vi "test grpc xnet.vi"() -> ()   [LabVIEW 2025]
uses:
  RPC Messages/nixnet_grpc_CreateSessionRequest.ctl
  RPC Messages/nixnet_grpc_CreateSessionRequest_mode_enum/nixnet_grpc_CreateSessionRequest_mode_enum.lvclass
  RPC Messages/nidevice_grpc_SessionInitializationBehavior.ctl
  RPC Messages/nixnet_grpc_CreateSessionMode.ctl
  RPC Messages/nixnet_grpc_CreateSessionRequest_mode_enum/nixnet_grpc_CreateSessionRequest_mode_enum.lvclass/nixnet_grpc_CreateSessionRequest_mode_enum.ctl
  RPC Messages/nixnet_grpc_ClearRequest.ctl
  RPC Messages/nidevice_grpc_Session.ctl
  RPC Messages/nixnet_grpc_SetPropertyRequest.ctl
  RPC Messages/nixnet_grpc_SetPropertyRequest_property_id_enum/nixnet_grpc_SetPropertyRequest_property_id_enum.lvclass
  RPC Messages/nixnet_grpc_SetPropertyRequest_property_value/nixnet_grpc_SetPropertyRequest_property_value.lvclass
  RPC Messages/nixnet_grpc_Property.ctl
  RPC Messages/nixnet_grpc_SetPropertyRequest_property_id_enum/nixnet_grpc_SetPropertyRequest_property_id_enum.lvclass/nixnet_grpc_SetPropertyRequest_property_id_enum.ctl
  RPC Messages/nixnet_grpc_SetPropertyRequest_property_value/nixnet_grpc_SetPropertyRequest_property_value.lvclass/nixnet_grpc_SetPropertyRequest_property_value.ctl
  RPC Messages/nixnet_grpc_ReadFrameRequest.ctl
  RPC Messages/nixnet_grpc_ReadFrameRequest_protocol_enum/nixnet_grpc_ReadFrameRequest_protocol_enum.lvclass
  RPC Messages/nixnet_grpc_ReadFrameRequest_timeout_enum/nixnet_grpc_ReadFrameRequest_timeout_enum.lvclass
  RPC Messages/nixnet_grpc_Protocol.ctl
  RPC Messages/nixnet_grpc_ReadFrameRequest_protocol_enum/nixnet_grpc_ReadFrameRequest_protocol_enum.lvclass/nixnet_grpc_ReadFrameRequest_protocol_enum.ctl
  RPC Messages/nixnet_grpc_TimeOut.ctl
  RPC Messages/nixnet_grpc_ReadFrameRequest_timeout_enum/nixnet_grpc_ReadFrameRequest_timeout_enum.lvclass/nixnet_grpc_ReadFrameRequest_timeout_enum.ctl
  RPC Messages/nixnet_grpc_FrameBufferResponse_frame/nixnet_grpc_FrameBufferResponse_frame.lvclass/nixnet_grpc_FrameBufferResponse_frame.ctl
  xnet-grpc_client.lvlib
  RPC Messages/nixnet_grpc_FrameBufferResponse_frame/nixnet_grpc_FrameBufferResponse_frame.lvclass
panel:
  out "new_session_initialized":bool
  out "create session status":i32
  out "status":i32
  out "payload":u8[](array[numeric])
  out "identifier":u32
  in  "Stop":bool
  out "error out":errorcluster
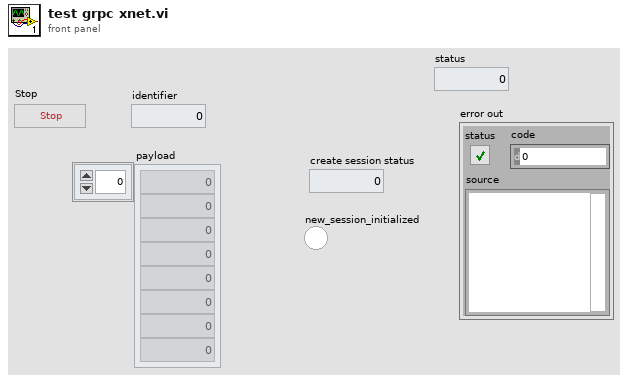
[diagram p1: front panel]
types:
  T1 = typedef "xnet-grpc_client.lvlib/nixnet_grpc_TimeOut.ctl" = enum32{"TIME_OUT_NONE", "TIME_OUT_INFINITE"}
  T2 = typedef "xnet-grpc_client.lvlib/nixnet_grpc_Protocol.ctl" = enum32{"PROTOCOL_UNSPECIFIED", "PROTOCOL_CAN", "PROTOCOL_LIN", "PROTOCOL_FLEX_RAY", "PROTOCOL_J1939", "PROTOCOL_ENET"}
  T3 = typedef "xnet-grpc_client.lvlib/nixnet_grpc_ReadFrameRequest.ctl" = cluster{"session":T4, "number_of_frames":i32, "max_payload_per_frame":u32, "nixnet_grpc_ReadFrameRequest_protocol_enum":refnum<class "nixnet_grpc_ReadFrameRequest_protocol_enum.lvclass">, "nixnet_grpc_ReadFrameRequest_timeout_enum":refnum<class "nixnet_grpc_ReadFrameRequest_timeout_enum.lvclass">}
  T4 = typedef "xnet-grpc_client.lvlib/nidevice_grpc_Session.ctl" = cluster{"name":string}
  T5 = typedef "xnet-grpc_client.lvlib/nixnet_grpc_Property.ctl" = enum32{"PROPERTY_UNSPECIFIED", "PROPERTY_SESSION_APPLICATION_PROTOCOL", "PROPERTY_SESSION_AUTO_START", "PROPERTY_SESSION_CLUSTER_NAME", "PROPERTY_SESSION_DATABASE_NAME", "PROPERTY_SESSION_ENET_FRAME_FILTER", "PROPERTY_SESSION_ENET_LOG_ERROR", "PROPERTY_SESSION_ENET_LOG_FILE", "PROPERTY_SESSION_ENET_LOG_MODE", "PROPERTY_SESSION_ENET_LOG_ENABLE_MULTIPLE_FILES", "PROPERTY_SESSION_ENET_LOG_FILE_SIZE_THRESHOLD", "PROPERTY_SESSION_ENET_LOG_OPERATION", "PROPERTY_SESSION_ENET_NUM_FRAMES_RECEIVED", "PROPERTY_SESSION_ENET_SOURCE_MAC_ADDRESS_AUTO", "PROPERTY_SESSION_INTF_BAUD_RATE_64", "PROPERTY_SESSION_INTF_ADJUST_LOCAL_TIME", "PROPERTY_SESSION_INTF_BAUD_RATE", "PROPERTY_SESSION_INTF_BUS_ERR_TO_IN_STRM", "PROPERTY_SESSION_INTF_CAN_FD_BAUD_RATE_64", "PROPERTY_SESSION_INTF_CAN_DISABLE_PROT_EXCEPTION_HANDLING", "PROPERTY_SESSION_INTF_CAN_EDGE_FILTER", "PROPERTY_SESSION_INTF_CAN_EXT_TCVR_CONFIG", "PROPERTY_SESSION_INTF_CAN_FD_BAUD_RATE", "PROPERTY_SESSION_INTF_CAN_FD_ISO_MODE", "PROPERTY_SESSION_INTF_CAN_IO_MODE", "PROPERTY_SESSION_INTF_CAN_LSTN_ONLY", "PROPERTY_SESSION_INTF_CAN_PEND_TX_ORDER", "PROPERTY_SESSION_INTF_CAN_SING_SHOT", "PROPERTY_SESSION_INTF_CAN_TERM", "PROPERTY_SESSION_INTF_CAN_TCVR_STATE", "PROPERTY_SESSION_INTF_CAN_TCVR_TYPE", "PROPERTY_SESSION_INTF_CAN_TX_IO_MODE", "PROPERTY_SESSION_INTF_CAN_TRANSMIT_PAUSE", "PROPERTY_SESSION_INTF_ECHO_TX", "PROPERTY_SESSION_INTF_ENET_EPT_RECEIVE_FILTER", "PROPERTY_SESSION_INTF_ENET_EPT_TRANSMIT_BANDWIDTH", "PROPERTY_SESSION_INTF_ENET_IPV4_ADDRESS", "PROPERTY_SESSION_INTF_ENET_JUMBO_FRAMES", "PROPERTY_SESSION_INTF_ENET_LINK_SPEED", "PROPERTY_SESSION_INTF_ENET_LINK_SPEED_CONFIGURED", "PROPERTY_SESSION_INTF_ENET_MAC_ADDRESS", "PROPERTY_SESSION_INTF_ENET_OS_NETWORK_ADAPTER_DESCRIPTION", "PROPERTY_SESSION_INTF_ENET_OS_NETWORK_ADAPTER_NAME", "PROPERTY_SESSION_INTF_ENET_OPERATIONAL_STATUS", "PROPERTY_SESSION_INTF_ENET_OUT_STRM_TIMESCALE", "PROPERTY_SESSION_INTF_ENET_PHY_POWER_MODE", "PROPERTY_SESSION_INTF_ENET_PHY_STATE", "PROPERTY_SESSION_INTF_ENET_PORT_MODE", "PROPERTY_SESSION_INTF_ENET_SIGNAL_QUALITY", "PROPERTY_SESSION_INTF_ENET_SLEEP_CAPABILITY", "PROPERTY_SESSION_INTF_ENET_STATS_COUNTER_NAMES", "PROPERTY_SESSION_INTF_ENET_STATS_COUNTER_VALUES", "PROPERTY_SESSION_INTF_ENET_STATS_RX_BAD_FRAMES", "PROPERTY_SESSION_INTF_ENET_STATS_RX_BYTES", "PROPERTY_SESSION_INTF_ENET_STATS_RX_GOOD_FRAMES", "PROPERTY_SESSION_INTF_ENET_STATS_TX_BYTES", "PROPERTY_SESSION_INTF_ENET_STATS_TX_GOOD_FRAMES", "PROPERTY_SESSION_INTF_ENET_STATS_PHY_COUNTER_NAMES", "PROPERTY_SESSION_INTF_ENET_STATS_PHY_COUNTER_VALUES", "PROPERTY_SESSION_INTF_ENET_STATS_PHY_LOW_POWER_SLEEP", "PROPERTY_SESSION_INTF_ENET_STATS_PHY_SLEEP_FAILURE", "PROPERTY_SESSION_INTF_ENET_STATS_PHY_WAKEUP_FAILURE", "PROPERTY_SESSION_INTF_ENET_STATS_PHY_WAKEUP_PULSE", "PROPERTY_SESSION_INTF_ENET_STATS_PHY_WAKEUP_REQUEST", "PROPERTY_SESSION_INTF_ENET_TIME_ADJUST_NETWORK_TIME", "PROPERTY_SESSION_INTF_ENET_TIME_BMCA_ENABLED", "PROPERTY_SESSION_INTF_ENET_TIME_CLK_ACCURACY", "PROPERTY_SESSION_INTF_ENET_TIME_CLK_CLASS", "PROPERTY_SESSION_INTF_ENET_TIME_CLK_ID", "PROPERTY_SESSION_INTF_ENET_TIME_CLK_OFFSET_VAR", "PROPERTY_SESSION_INTF_ENET_TIME_GM_CLK_ACCURACY", "PROPERTY_SESSION_INTF_ENET_TIME_GM_CLK_CLASS", "PROPERTY_SESSION_INTF_ENET_TIME_GM_CLK_ID", "PROPERTY_SESSION_INTF_ENET_TIME_GM_CLK_OFFSET_VAR", "PROPERTY_SESSION_INTF_ENET_TIME_GM_PRIORITY_1", "PROPERTY_SESSION_INTF_ENET_TIME_GM_PRIORITY_2", "PROPERTY_SESSION_INTF_ENET_TIME_OFFSET_FROM_MASTER", "PROPERTY_SESSION_INTF_ENET_TIME_PORT_AS_CAPABLE", "PROPERTY_SESSION_INTF_ENET_TIME_PORT_ANNOUNCE_RECEIPT_TIMEOUT", "PROPERTY_SESSION_INTF_ENET_TIME_PORT_ANNOUNCE_TRANSMIT_ENABLED", "PROPERTY_SESSION_INTF_ENET_TIME_PORT_LOG_ANNOUNCE_INTERVAL", "PROPERTY_SESSION_INTF_ENET_TIME_PORT_LOG_ANNOUNCE_INTERVAL_CONFIGURED", "PROPERTY_SESSION_INTF_ENET_TIME_PORT_LOG_PDELAY_INTERVAL", "PROPERTY_SESSION_INTF_ENET_TIME_PORT_LOG_PDELAY_INTERVAL_CONFIGURED", "PROPERTY_SESSION_INTF_ENET_TIME_PORT_LOG_SYNC_INTERVAL", "PROPERTY_SESSION_INTF_ENET_TIME_PORT_LOG_SYNC_INTERVAL_CONFIGURED", "PROPERTY_SESSION_INTF_ENET_TIME_PORT_PDELAY_ENABLED", "PROPERTY_SESSION_INTF_ENET_TIME_PORT_STATE", "PROPERTY_SESSION_INTF_ENET_TIME_PORT_STATE_CONFIGURED", "PROPERTY_SESSION_INTF_ENET_TIME_PORT_PROP_DELAY", "PROPERTY_SESSION_INTF_ENET_TIME_PORT_PROP_DELAY_CONFIGURED", "PROPERTY_SESSION_INTF_ENET_TIME_PORT_PROP_DELAY_THRESHOLD", "PROPERTY_SESSION_INTF_ENET_TIME_PORT_STATS_COUNTER_NAMES", "PROPERTY_SESSION_INTF_ENET_TIME_PORT_STATS_COUNTER_VALUES", "PROPERTY_SESSION_INTF_ENET_TIME_PORT_STATS_RX_ANNOUNCE", "PROPERTY_SESSION_INTF_ENET_TIME_PORT_STATS_RX_PDELAY_REQUEST", "PROPERTY_SESSION_INTF_ENET_TIME_PORT_STATS_RX_SYNC", "PROPERTY_SESSION_INTF_ENET_TIME_PORT_STATS_TX_ANNOUNCE", "PROPERTY_SESSION_INTF_ENET_TIME_PORT_STATS_TX_PDELAY_REQUEST", "PROPERTY_SESSION_INTF_ENET_TIME_PORT_STATS_TX_SYNC", "PROPERTY_SESSION_INTF_ENET_TIME_PORT_SYNC_RECEIPT_TIMEOUT", "PROPERTY_SESSION_INTF_ENET_TIME_PORT_SYNC_STATUS", "PROPERTY_SESSION_INTF_ENET_TIME_PORT_SYNCED", "PROPERTY_SESSION_INTF_ENET_TIME_PRIORITY_1", "PROPERTY_SESSION_INTF_ENET_TIME_PRIORITY_2", "PROPERTY_SESSION_INTF_ENET_TIME_PROTOCOL", "PROPERTY_SESSION_INTF_ENET_TIME_PROTOCOL_ENABLED", "PROPERTY_SESSION_INTF_ENET_TIME_STEPS_TO_GM", "PROPERTY_SESSION_INTF_ENET_TRIGGER_PPS_SYNCED", "PROPERTY_SESSION_INTF_FLEX_RAY_ACC_START_RNG", "PROPERTY_SESSION_INTF_FLEX_RAY_ALW_HLT_CLK", "PROPERTY_SESSION_INTF_FLEX_RAY_ALW_PASS_ACT", "PROPERTY_SESSION_INTF_FLEX_RAY_AUTO_ASLP_WHN_STP", "PROPERTY_SESSION_INTF_FLEX_RAY_CLST_DRIFT_DMP", "PROPERTY_SESSION_INTF_FLEX_RAY_COLDSTART", "PROPERTY_SESSION_INTF_FLEX_RAY_CONNECTED_CHS", "PROPERTY_SESSION_INTF_FLEX_RAY_DEC_CORR", "PROPERTY_SESSION_INTF_FLEX_RAY_DELAY_COMP_A", "PROPERTY_SESSION_INTF_FLEX_RAY_DELAY_COMP_B", "PROPERTY_SESSION_INTF_FLEX_RAY_KEY_SLOT_ID", "PROPERTY_SESSION_INTF_FLEX_RAY_LATEST_TX", "PROPERTY_SESSION_INTF_FLEX_RAY_LIST_TIMO", "PROPERTY_SESSION_INTF_FLEX_RAY_MAC_INIT_OFF_A", "PROPERTY_SESSION_INTF_FLEX_RAY_MAC_INIT_OFF_B", "PROPERTY_SESSION_INTF_FLEX_RAY_MAX_DRIFT", "PROPERTY_SESSION_INTF_FLEX_RAY_MIC_INIT_OFF_A", "PROPERTY_SESSION_INTF_FLEX_RAY_MIC_INIT_OFF_B", "PROPERTY_SESSION_INTF_FLEX_RAY_MICROTICK", "PROPERTY_SESSION_INTF_FLEX_RAY_NULL_TO_IN_STRM", "PROPERTY_SESSION_INTF_FLEX_RAY_OFF_CORR", "PROPERTY_SESSION_INTF_FLEX_RAY_OFF_CORR_OUT", "PROPERTY_SESSION_INTF_FLEX_RAY_RATE_CORR", "PROPERTY_SESSION_INTF_FLEX_RAY_RATE_CORR_OUT", "PROPERTY_SESSION_INTF_FLEX_RAY_SAMP_PER_MICRO", "PROPERTY_SESSION_INTF_FLEX_RAY_SING_SLOT_EN", "PROPERTY_SESSION_INTF_FLEX_RAY_SLEEP", "PROPERTY_SESSION_INTF_FLEX_RAY_STATISTICS_EN", "PROPERTY_SESSION_INTF_FLEX_RAY_SYM_TO_IN_STRM", "PROPERTY_SESSION_INTF_FLEX_RAY_SYNC_STATUS", "PROPERTY_SESSION_INTF_FLEX_RAY_SYNC_CH_A_EVEN", "PROPERTY_SESSION_INTF_FLEX_RAY_SYNC_CH_A_ODD", "PROPERTY_SESSION_INTF_FLEX_RAY_SYNC_CH_B_EVEN", "PROPERTY_SESSION_INTF_FLEX_RAY_SYNC_CH_B_ODD", "PROPERTY_SESSION_INTF_FLEX_RAY_TERM", "PROPERTY_SESSION_INTF_FLEX_RAY_WAKEUP_CH", "PROPERTY_SESSION_INTF_FLEX_RAY_WAKEUP_PTRN", "PROPERTY_SESSION_INTF_NAME", "PROPERTY_SESSION_INTF_LIN_BREAK_DELIMITER_LENGTH", "PROPERTY_SESSION_INTF_LIN_BREAK_LENGTH", "PROPERTY_SESSION_INTF_LIN_CHECKSUM_TO_IN_STRM", "PROPERTY_SESSION_INTF_LIN_DIAG_P2_MIN", "PROPERTY_SESSION_INTF_LIN_DIAG_ST_MIN", "PROPERTY_SESSION_INTF_LIN_MASTER", "PROPERTY_SESSION_INTF_LIN_NO_RESPONSE_TO_IN_STRM", "PROPERTY_SESSION_INTF_LINO_STR_SLV_RSP_LST_BY_NAD", "PROPERTY_SESSION_INTF_LIN_SCHED_NAMES", "PROPERTY_SESSION_INTF_LIN_SLEEP", "PROPERTY_SESSION_INTF_LIN_ALW_START_WO_BUS_PWR", "PROPERTY_SESSION_INTF_LIN_TERM", "PROPERTY_SESSION_INTF_OUT_STRM_LIST", "PROPERTY_SESSION_INTF_OUT_STRM_LIST_BY_ID", "PROPERTY_SESSION_INTF_OUT_STRM_TIMNG", "PROPERTY_SESSION_INTF_SRC_TERM_START_TRIGGER", "PROPERTY_SESSION_INTF_START_TRIG_TO_IN_STRM", "PROPERTY_SESSION_LIST", "PROPERTY_SESSION_MODE", "PROPERTY_SESSION_NUM_IN_LIST", "PROPERTY_SESSION_NUM_FRAMES", "PROPERTY_SESSION_NUM_PEND", "PROPERTY_SESSION_NUM_UNUSED", "PROPERTY_SESSION_PAYLD_LEN_MAX", "PROPERTY_SESSION_PROTOCOL", "PROPERTY_SESSION_QUEUE_SIZE", "PROPERTY_SESSION_RESAMP_RATE", "PROPERTY_SESSION_J1939_ECU", "PROPERTY_SESSION_J1939_ECU_BUSY", "PROPERTY_SESSION_J1939_FILL_BYTE", "PROPERTY_SESSION_J1939_INCLUDE_DEST_ADDR_IN_PGN", "PROPERTY_SESSION_J1939_MAX_REPEAT_CTS", "PROPERTY_SESSION_J1939_ADDRESS", "PROPERTY_SESSION_J1939_NAME", "PROPERTY_SESSION_J1939_NUM_PACKETS_RECV", "PROPERTY_SESSION_J1939_NUM_PACKETS_RESP", "PROPERTY_SESSION_J1939_HOLD_TIME_TH", "PROPERTY_SESSION_J1939_RESPONSE_TIME_TR_GD", "PROPERTY_SESSION_J1939_RESPONSE_TIME_TR_SD", "PROPERTY_SESSION_J1939_TIMEOUT_T1", "PROPERTY_SESSION_J1939_TIMEOUT_T2", "PROPERTY_SESSION_J1939_TIMEOUT_T3", "PROPERTY_SESSION_J1939_TIMEOUT_T4", "PROPERTY_SESSION_J1939_WRITE_QUEUE_SIZE", "PROPERTY_SYS_CDAQ_PKT_TIME", "PROPERTY_SYS_DEV_REFS", "PROPERTY_SYS_INTF_REFS", "PROPERTY_SYS_INTF_REFS_ALL", "PROPERTY_SYS_INTF_REFS_CAN", "PROPERTY_SYS_INTF_REFS_ETHERNET", "PROPERTY_SYS_INTF_REFS_FLEX_RAY", "PROPERTY_SYS_INTF_REFS_LIN", "PROPERTY_SYS_VER_BUILD", "PROPERTY_SYS_VER_MAJOR", "PROPERTY_SYS_VER_MINOR", "PROPERTY_SYS_VER_PHASE", "PROPERTY_SYS_VER_UPDATE", "PROPERTY_DEV_FORM_FAC", "PROPERTY_DEV_INTF_REFS", "PROPERTY_DEV_INTF_REFS_ALL", "PROPERTY_DEV_NUM_PORTS", "PROPERTY_DEV_NUM_PORTS_ALL", "PROPERTY_DEV_NAME", "PROPERTY_DEV_PRODUCT_NUM", "PROPERTY_DEV_SER_NUM", "PROPERTY_DEV_SLOT_NUM", "PROPERTY_INTF_CAN_TERM_CAP", "PROPERTY_INTF_CAN_TCVR_CAP", "PROPERTY_INTF_DEV_REF", "PROPERTY_INTF_DONGLE_COMPATIBLE_FIRMWARE_VERSION", "PROPERTY_INTF_DONGLE_COMPATIBLE_REVISION", "PROPERTY_INTF_DONGLE_FIRMWARE_VERSION", "PROPERTY_INTF_DONGLE_ID", "PROPERTY_INTF_DONGLE_REVISION", "PROPERTY_INTF_DONGLE_STATE", "PROPERTY_INTF_NAME", "PROPERTY_INTF_NUM", "PROPERTY_INTF_PORT_NUM", "PROPERTY_INTF_PROTOCOL"}
  T6 = typedef "xnet-grpc_client.lvlib/nixnet_grpc_SetPropertyRequest.ctl" = cluster{"session":T4, "nixnet_grpc_SetPropertyRequest_property_id_enum":refnum<class "nixnet_grpc_SetPropertyRequest_property_id_enum.lvclass">, "nixnet_grpc_SetPropertyRequest_property_value":refnum<class "nixnet_grpc_SetPropertyRequest_property_value.lvclass">}
  T7 = typedef "xnet-grpc_client.lvlib/nixnet_grpc_ClearRequest.ctl" = cluster{"session":T4}
  T8 = typedef "xnet-grpc_client.lvlib/nidevice_grpc_SessionInitializationBehavior.ctl" = enum32{"SESSION_INITIALIZATION_BEHAVIOR_UNSPECIFIED", "SESSION_INITIALIZATION_BEHAVIOR_INITIALIZE_NEW", "SESSION_INITIALIZATION_BEHAVIOR_ATTACH_TO_EXISTING"}
  T9 = typedef "xnet-grpc_client.lvlib/nixnet_grpc_CreateSessionMode.ctl" = enum32{"CREATE_SESSION_MODE_SIGNAL_IN_SINGLE_POINT", "CREATE_SESSION_MODE_SIGNAL_IN_WAVEFORM", "CREATE_SESSION_MODE_SIGNAL_IN_XY", "CREATE_SESSION_MODE_SIGNAL_OUT_SINGLE_POINT", "CREATE_SESSION_MODE_SIGNAL_OUT_WAVEFORM", "CREATE_SESSION_MODE_SIGNAL_OUT_XY", "CREATE_SESSION_MODE_FRAME_IN_STREAM", "CREATE_SESSION_MODE_FRAME_IN_QUEUED", "CREATE_SESSION_MODE_FRAME_IN_SINGLE_POINT", "CREATE_SESSION_MODE_FRAME_OUT_STREAM", "CREATE_SESSION_MODE_FRAME_OUT_QUEUED", "CREATE_SESSION_MODE_FRAME_OUT_SINGLE_POINT", "CREATE_SESSION_MODE_SIGNAL_CONVERSION_SINGLE_POINT"}
  T10 = typedef "xnet-grpc_client.lvlib/nixnet_grpc_CreateSessionRequest.ctl" = cluster{"session_name":string, "database_name":string, "cluster_name":string, "list":string, "interface_name":string, "CreateSessionRequest_mode_enum":refnum<class "nixnet_grpc_CreateSessionRequest_mode_enum.lvclass">, "initialization_behavior":T8}
  T11 = typedef "grpc-lvsupport-release.lvlib/grpcId.ctl" = u64
  T12 = typedef "xnet-grpc_client.lvlib/nixnet_grpc_CreateSessionResponse.ctl" = cluster{"status":i32, "session":T4, "new_session_initialized":bool}
  T13 = typedef "xnet-grpc_client.lvlib/nixnet_grpc_ReadFrameResponse.ctl" = cluster{"status":i32, "buffer":T14[]}
  T14 = typedef "xnet-grpc_client.lvlib/nixnet_grpc_FrameBufferResponse.ctl" = cluster{"nixnet_grpc_FrameBufferResponse_frame":refnum<class "nixnet_grpc_FrameBufferResponse_frame.lvclass">}
  T15 = typedef "xnet-grpc_client.lvlib/nixnet_grpc_FrameResponse.ctl" = cluster{"timestamp":u64, "identifier":u32, "type":T16, "type_raw":u32, "flags":T17[], "flags_raw":u32, "info":u32, "payload":u8[]}
  T16 = typedef "xnet-grpc_client.lvlib/nixnet_grpc_FrameType.ctl" = enum32{"FRAME_TYPE_CAN_DATA", "FRAME_TYPE_CAN_REMOTE", "FRAME_TYPE_CAN_BUS_ERROR", "FRAME_TYPE_CAN20_DATA", "FRAME_TYPE_CANFD_DATA", "FRAME_TYPE_CANFDBRS_DATA", "FRAME_TYPE_FLEX_RAY_DATA", "FRAME_TYPE_FLEX_RAY_NULL", "FRAME_TYPE_FLEX_RAY_SYMBOL", "FRAME_TYPE_LIN_DATA", "FRAME_TYPE_LIN_BUS_ERROR", "FRAME_TYPE_LIN_NO_RESPONSE", "FRAME_TYPE_J1939_DATA", "FRAME_TYPE_SPECIAL_DELAY", "FRAME_TYPE_SPECIAL_LOG_TRIGGER", "FRAME_TYPE_SPECIAL_START_TRIGGER"}
  T17 = typedef "xnet-grpc_client.lvlib/nixnet_grpc_FrameFlags.ctl" = enum32{"FRAME_FLAGS_UNSPECIFIED", "FRAME_FLAGS_FLEX_RAY_STARTUP", "FRAME_FLAGS_FLEX_RAY_SYNC", "FRAME_FLAGS_FLEX_RAY_PREAMBLE", "FRAME_FLAGS_FLEX_RAY_CH_A", "FRAME_FLAGS_FLEX_RAY_CH_B", "FRAME_FLAGS_LIN_EVENT_SLOT", "FRAME_FLAGS_TRANSMIT_ECHO"}
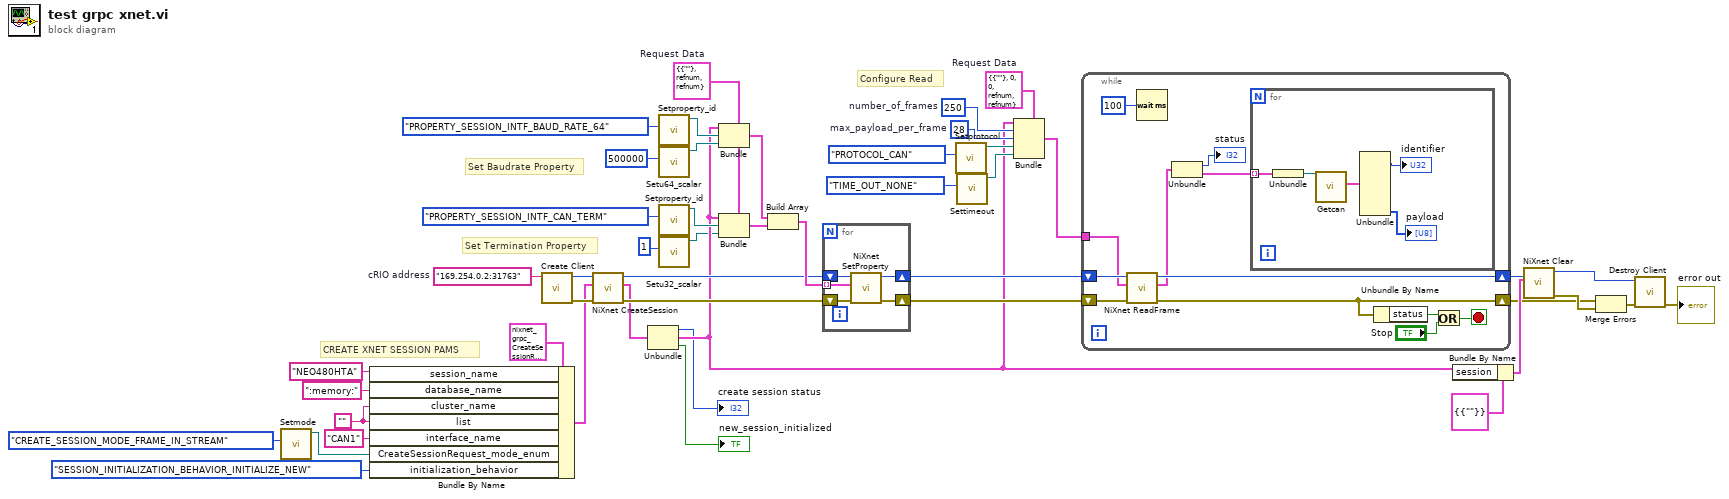
[diagram p0: block diagram]
diagram:
  w7 = u32 28  # max_payload_per_frame
  w10 = 250  # number_of_frames
  w17 = T3 {"session"={"name"=""}, "number_of_frames"=0, "max_payload_per_frame"=0, "nixnet_grpc_ReadFrameRequest_protocol_enum"=refnum, "nixnet_grpc_ReadFrameRequest_timeout_enum"=refnum}  # Request Data
  w27 = T6 {"session"={"name"=""}, "nixnet_grpc_SetPropertyRequest_property_id_enum"=refnum, "nixnet_grpc_SetPropertyRequest_property_value"=refnum}  # Request Data
  w6 = ""
  w48 = "169.254.0.2:31763"  # cRIO address
  # "CREATE XNET SESSION PAMS"
  # "Configure Read"
  # "Set Termination Property"
  # "Set Baudrate Property"
  n1 = call "Setmode.vi"("Set_Val"=nixnet_grpc_CreateSessionMode."CREATE_SESSION_MODE_FRAME_IN_STREAM") -> ("OneOfTemplate out"=w40:refnum<class "nixnet_grpc_CreateSessionRequest_mode_enum.lvclass">)  [unwired: 10 in]
  n2 = Bundle By Name(cluster=T10 {"session_name"="", "database_name"="", "cluster_name"="", "list"="", "interface_name"="", "CreateSessionRequest_mode_enum"=refnum, "initialization_behavior"=enum."SESSION_INITIALIZATION_BEHAVIOR_UNSPECIFIED"} ("Request Data"), "session_name"="NEO480HTA", "database_name"=":memory:", "cluster_name"=w6, "list"=w6, "interface_name"="CAN1", "CreateSessionRequest_mode_enum"=w40, "initialization_behavior"=nidevice_grpc_SessionInitializationBehavior."SESSION_INITIALIZATION_BEHAVIOR_INITIALIZE_NEW") -> (w38:T10)
  n3 = call "Create Client.vi"("address"=w48) -> ("error out"=w46:errorcluster, "gRPC ID Out"=w44:T11)  [unwired: 9 in]
  n4 = call "NiXnet CreateSession.vi"("error in"=w46, "Request Data"=w38, "gRPC ID"=w44) -> ("error out"=w45:errorcluster, "Response Data"=w31:T12, "gRPC ID out"=w9:T11)  [unwired: 6 in]
  n5 = Unbundle(w31) -> ("status"=→"create session status":i32, "session"=w5:T4, "new_session_initialized"=→"new_session_initialized":bool)
  n6 = call "Setproperty_id.vi"("Set_Val"=nixnet_grpc_Property."PROPERTY_SESSION_INTF_BAUD_RATE_64") -> ("OneOfTemplate out"=w26:refnum<class "nixnet_grpc_SetPropertyRequest_property_id_enum.lvclass">)  [unwired: 10 in]
  n7 = call "Setu64_scalar.vi"("Set_Val"=u64 500000) -> ("OneOfTemplate out"=w25:refnum<class "nixnet_grpc_SetPropertyRequest_property_value.lvclass">)  [unwired: 10 in]
  n8 = call "Setproperty_id.vi"("Set_Val"=nixnet_grpc_Property."PROPERTY_SESSION_INTF_CAN_TERM") -> ("OneOfTemplate out"=w22:refnum<class "nixnet_grpc_SetPropertyRequest_property_id_enum.lvclass">)  [unwired: 10 in]
  n9 = call "Setu32_scalar.vi"("Set_Val"=u32 1) -> ("OneOfTemplate out"=w1:refnum<class "nixnet_grpc_SetPropertyRequest_property_value.lvclass">)  [unwired: 10 in]
  n10 = Bundle(cluster=w27, "session"=w5, "nixnet_grpc_SetPropertyRequest_property_id_enum"=w26, "nixnet_grpc_SetPropertyRequest_property_value"=w25) -> (w20:T6)
  n11 = Bundle(cluster=w27, "session"=w5, "nixnet_grpc_SetPropertyRequest_property_id_enum"=w22, "nixnet_grpc_SetPropertyRequest_property_value"=w1) -> (w28:T6)
  n12 = Build Array(w20, w28) -> (w21:T6[])
  n13 = for {
    tunnel: w21 -> [w50] mode=indexing
    shift-right: [w52] -> w19
    shift-left: w45 -> [w53]
    shift-right: [w49] -> w8
    shift-left: w9 -> [w51]
    n14 = call "NiXnet SetProperty.vi"("error in"=w53, "Request Data"=w50, "gRPC ID"=w51) -> ("error out"=w52:errorcluster, "gRPC ID out"=w49:T11)  [unwired: 6 in, 1 out]
  }
  n15 = call "Setprotocol.vi"("Set_Val"=nixnet_grpc_Protocol."PROTOCOL_CAN") -> ("OneOfTemplate out"=w14:refnum<class "nixnet_grpc_ReadFrameRequest_protocol_enum.lvclass">)  [unwired: 10 in]
  n16 = call "Settimeout.vi"("Set_Val"=nixnet_grpc_TimeOut."TIME_OUT_NONE") -> ("OneOfTemplate out"=w12:refnum<class "nixnet_grpc_ReadFrameRequest_timeout_enum.lvclass">)  [unwired: 10 in]
  n17 = Bundle(cluster=w17, "session"=w5, "number_of_frames"=w10, "max_payload_per_frame"=w7, "nixnet_grpc_ReadFrameRequest_protocol_enum"=w14, "nixnet_grpc_ReadFrameRequest_timeout_enum"=w12) -> (w16:T3)
  n18 = while {
    shift-right: [w63] -> w18
    shift-left: w8 -> [w65]
    shift-right: [w58] -> w13
    shift-left: w19 -> [w64]
    tunnel: w16 -> [w62]
    stop <- w59 stop-if-true
    n19 = call "NiXnet ReadFrame.vi"("error in"=w64, "Request Data"=w62, "gRPC ID"=w65) -> ("error out"=w58:errorcluster, "Response Data"=w61:T13, "gRPC ID out"=w63:T11)  [unwired: 6 in]
    n20 = Wait (ms)(milliseconds to wait=u32 100) -> ()  [unwired: 1 out]
    n21 = Unbundle(w61) -> ("status"=→"status":i32, "buffer"=w60:T14[])
    n22 = for {
      tunnel: w60 -> [w70] mode=indexing
      n23 = Unbundle(w70) -> ("nixnet_grpc_FrameBufferResponse_frame"=w66:refnum<class "nixnet_grpc_FrameBufferResponse_frame.lvclass">)
      n24 = call "Getcan.vi"("OneOfTemplate in"=w66) -> ("Get_Val"=w69:T15)  [unwired: 9 in, 1 out]
      n25 = Unbundle(w69) -> ("identifier"=→"identifier":u32, "payload"=→"payload":u8[])  [unwired: 6 out]
    }
    n26 = Unbundle By Name(w58) -> ("status"=w56:bool)
    n27 = Or(x=w56, y="Stop") -> (x .or. y?=w59:bool)
  }
  n28 = Bundle By Name(cluster=T7 {"session"={"name"=""}} ("Request Data"), "session"=w5) -> (w35:T7)
  n29 = call "NiXnet Clear.vi"("Request Data"=w35, "gRPC ID"=w18) -> ("error out"=w33:errorcluster, "gRPC ID out"=w37:T11)  [unwired: 7 in, 1 out]
  n30 = Merge Errors(w13, w33) -> (w34:errorcluster)
  n31 = call "Destroy Client.vi"("error in"=w34, "gRPC ID"=w37) -> ("error out"=→"error out":errorcluster)  [unwired: 9 in]
